vi "Thor Drive.vi"(9 "Gear 2":bool, 10 "Turn Power":dbl, 11 "Y Power":dbl) -> (1 "Gear 2":bool, 2 "Turn power":dbl, 3 "Y power":dbl)   [LabVIEW 2017]
panel:
  out "Brake":bool
  in  "Brake 2":bool
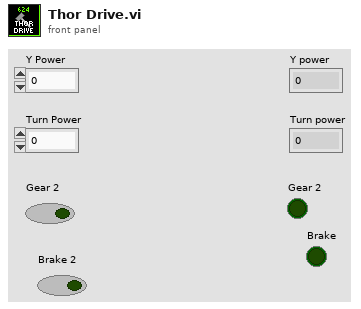
[diagram p1: front panel]
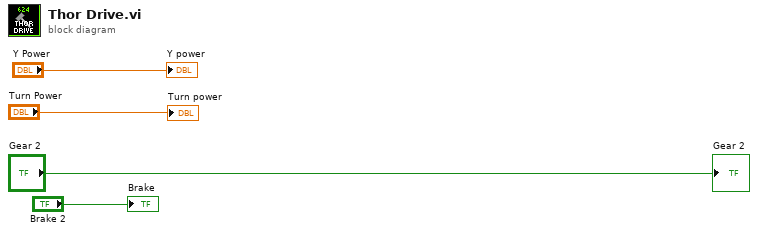
[diagram p0: block diagram]
diagram:
  "Y power" <- "Y Power"
  "Turn power" <- "Turn Power"
  "Gear 2" <- "Gear 2"
  "Brake" <- "Brake 2"
